vi "Close.vi"(8 "error in (no error)":errorcluster, 11 "VXMx2 in":refnum<class "VXMx2.lvclass">) -> (0 "error out":errorcluster, 3 "VXMx2 out":refnum<class "VXMx2.lvclass">)   [LabVIEW 2019, in "VXMx2.lvclass"]
uses:
  VXMx2.lvclass
  VXMx2.lvclass/VXMx2.ctl
  <instrlib>/Velmex VXM/Velmex VXM.lvlib
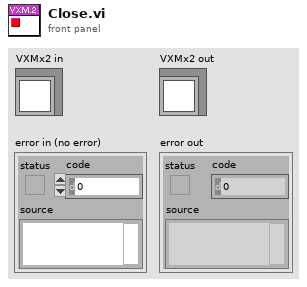
[diagram p1: front panel]
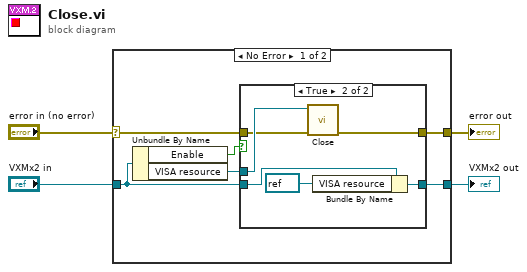
[diagram p0: block diagram]
diagram:
  n1 = case shown="No Error" "error in (no error)" {
    selector: "error in (no error)" -> [w6 w20]
    tunnel: [w5 w20] -> w3
    tunnel: [w7 w19] -> w1
    tunnel: "VXMx2 in" -> [w8 w19]
    frame No Error {
      n2 = Unbundle By Name(w8) -> ("Enable"=w10:bool, "VISA resource"=w9:refnum<visa-resource-name>)
      n3 = case shown="True" w10 {
        tunnel: w9 -> [_ w18]
        tunnel: [w12 w16] -> w7
        tunnel: w8 -> [w12 w17]
        tunnel: [w11 w14] -> w5
        tunnel: w6 -> [w11 w13]
        frame False {
        }
        frame True {
          n4 = call <instrlib>:"Close.vi"("error in (no error)"=w13, "VISA resource name"=w18) -> ("error out"=w14:errorcluster)  [unwired: 9 in]
          n5 = Bundle By Name(cluster=w17, "VISA resource"=refnum<visa-resource-name> refnum) -> (w16:refnum<class "VXMx2.lvclass">)
        }
      }
    }
    frame Error {
    }
  }
  "error out" <- w3
  "VXMx2 out" <- w1
